vi "AddPanel.vi"(8 "error in":errorcluster caption="错误输入（无错误）", 10 "Vi Alias":string, 11 "PanelRootNode 输入":refnum<class "PanelRootNode.lvclass"> caption="DNL_LabVIEW Object in") -> (0 "error out":errorcluster caption="错误输出", 3 "PanelRootNode 输出":refnum<class "PanelRootNode.lvclass"> caption="DNL_LabVIEW Object out")   [LabVIEW 2013, in "PanelRootNode.lvclass"]
uses:
  PanelRootNode.lvclass
  PanelDataNode/Split Mode.ctl
  PanelDataNode/PanelDataNode.lvclass
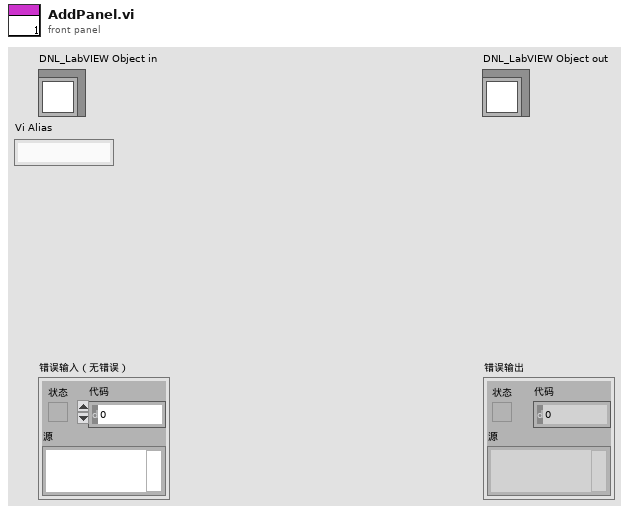
[diagram p1: front panel]
types:
  T1 = typedef "PanelDataNode.lvclass/Split Mode.ctl" = enum16{"Horizontal(up)", "Vertical(left)", "Horizontal(down)", "Vertical(right)"}
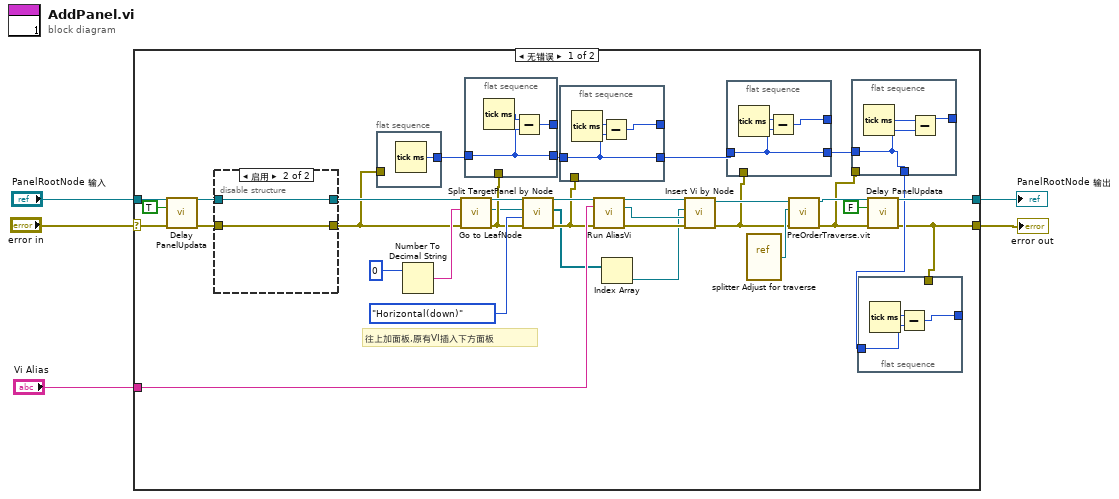
[diagram p0: block diagram]
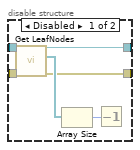
[diagram p2: hidden frame]
diagram:
  n1 = case shown="无错误" "error in" {
    selector: "error in" -> [w31 w65]
    tunnel: [w14 w65] -> w4
    tunnel: [w36 w64] -> w2
    tunnel: "PanelRootNode 输入" -> [w33 w64]
    tunnel: "Vi Alias" -> [w39 _]
    frame No Error {
      # "往上加面板,原有VI插入下方面板"
      n2 = call "Delay PanelUpdata.vi"("error in (no error)"=w31, "延迟前面板更新"=TRUE, "PanelRootNode 输入"=w33) -> ("error out"=w34:errorcluster, "PanelRootNode 输出"=w32:refnum<class "PanelRootNode.lvclass">)  [unwired: 7 in]
      n3 = disable-structure shown="启用" {
        disable-tunnel: [w60 w63] -> w38
        disable-tunnel: [w59 w62] -> w21
        disable-tunnel: w34 -> [w58 w62]
        disable-tunnel: w32 -> [w57 w63]
        frame Disabled {
          n4 = call-dynamic "Get LeafNodes.vi"("error in (no error)"=w58, "PanelRootNode 输入"=w57) -> ("error out"=w59:errorcluster, "DataNode[]"=w61:refnum<data-value>[], "PanelRootNode 输出"=w60:refnum<class "PanelRootNode.lvclass">)  [unwired: 7 in]
          n5 = Array Size(array=w61) -> (size(s)=w56:i32)
          n6 = Decrement(x=w56) -> ()  [unwired: 1 out]
        }
        frame Enabled {
        }
      }
      n7 = flat-sequence {
        tunnel: [w55] -> w23
        tunnel: w21 -> [_]
        frame #0 {
          n8 = Tick Count (ms)() -> (millisecond timer value=w55:u32)
        }
      }
      n9 = Number To Decimal String(number=0) -> (decimal integer string=w29:string)  [unwired: 1 in]
      n10 = call-dynamic "Go to LeafNode.vi"("error in"=w21, "LeafNumber"=w29, "PanelRootNode 输入"=w38) -> ("error out"=w20:errorcluster, "Node*"=w8:refnum<data-value>, "PanelRootNode 输出"=w27:refnum<class "PanelRootNode.lvclass">)  [unwired: 5 in, 1 out]
      n11 = flat-sequence {
        tunnel: [w53] -> w22
        tunnel: w23 -> [w53]
        tunnel: w20 -> [_]
        tunnel: [w52] -> _
        frame #0 {
          n12 = Tick Count (ms)() -> (millisecond timer value=w54:u32)
          n13 = Subtract(x=w54, y=w53) -> (x-y=w52:u32)
        }
      }
      n14 = call-dynamic "Split TargetPanel by Node.vi"("error in"=w20, "Split Mode"=Split_Mode."Horizontal(down)", "Node*"=w8, "PanelRootNode 输入"=w27) -> ("error out"=w19:errorcluster, "ChildDataNode[]"=w7:refnum<data-value>[], "PanelRootNode 输出"=w37:refnum<class "PanelRootNode.lvclass">)  [unwired: 5 in]
      n15 = flat-sequence {
        tunnel: w22 -> [w49]
        tunnel: w19 -> [_]
        tunnel: [w50] -> _
        tunnel: [w49] -> w18
        frame #0 {
          n16 = Tick Count (ms)() -> (millisecond timer value=w51:u32)
          n17 = Subtract(x=w51, y=w49) -> (x-y=w50:u32)
        }
      }
      n18 = call-dynamic "Run AliasVi.vi"("error in (no error)"=w19, "Vi Alias"=w39, "PanelDataNode 输入"=w37) -> ("error out"=w11:errorcluster, "VI*"=w9:refnum<vi>, "PanelDataNode 输出"=w13:refnum<class "PanelRootNode.lvclass">)  [unwired: 6 in]
      n19 = Index Array(array=w7) -> (element=w6:refnum<data-value>)  [unwired: 1 in]
      n20 = call-dynamic "Insert Vi by Node.vi"("error in"=w11, "dynamic VI*"=w9, "Node*"=w6, "PanelRootNode 输入"=w13) -> ("error out"=w10:errorcluster, "PanelRootNode 输出"=w12:refnum<class "PanelRootNode.lvclass">)  [unwired: 6 in]
      n21 = flat-sequence {
        tunnel: w18 -> [w46]
        tunnel: [w47] -> _
        tunnel: w10 -> [_]
        tunnel: [w46] -> w17
        frame #0 {
          n22 = Tick Count (ms)() -> (millisecond timer value=w48:u32)
          n23 = Subtract(x=w48, y=w46) -> (x-y=w47:u32)
        }
      }
      n24 = vi-ref "splitter Adjust for traverse.vi"() -> (w25:refnum<vi>)
      n25 = call-dynamic "PreOrderTraverse.vit"("error in"=w10, "vi reference"=w25, "PanelLinkNode 输入"=w12) -> ("error out"=w16:errorcluster, "PanelLinkNode 输出"=w26:refnum<class "PanelRootNode.lvclass">)  [unwired: 5 in, 2 out]
      n26 = flat-sequence {
        tunnel: w17 -> [w43]
        tunnel: [w44] -> _
        tunnel: w16 -> [_]
        tunnel: [w43] -> w15
        frame #0 {
          n27 = Tick Count (ms)() -> (millisecond timer value=w45:u32)
          n28 = Subtract(x=w45, y=w43) -> (x-y=w44:u32)
        }
      }
      n29 = flat-sequence {
        tunnel: w15 -> [w41]
        tunnel: [w40] -> _
        tunnel: w14 -> [_]
        frame #0 {
          n30 = Tick Count (ms)() -> (millisecond timer value=w42:u32)
          n31 = Subtract(x=w42, y=w41) -> (x-y=w40:u32)
        }
      }
      n32 = call "Delay PanelUpdata.vi"("error in (no error)"=w16, "延迟前面板更新"=FALSE, "PanelRootNode 输入"=w26) -> ("error out"=w14:errorcluster, "PanelRootNode 输出"=w36:refnum<class "PanelRootNode.lvclass">)  [unwired: 7 in]
    }
    frame Error {
    }
  }
  "error out" <- w4
  "PanelRootNode 输出" <- w2
